vi "Save-Load General Setup Parameters.vi"(8 "error in":errorcluster, 11 "Function":T1=enum."Load from file") -> (0 "error out":errorcluster)   [LabVIEW 2013]
uses:
  Typedefs/Save-Load enum.ctl
  Typedefs/Which path.ctl
  <vilib>/Utility/config.llb/NI_LVConfig.lvlib
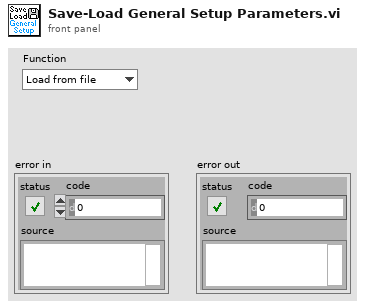
[diagram p1: front panel]
types:
  T1 = typedef "Save-Load enum.ctl" = enum16{"Save to file", "Load from file", "Compare from file"}
  T2 = typedef "Which path.ctl" = enum16{"Configuration Files", "Calibration Files", "Images", "Setup.ini", "Loaded User profile.ini", "User's-Previous session.ini", "New user profile.ini", "Selected User profile.ini", "User profiles folder", "Power meter scaling.txt", "FOV Cal.ini"}
  T3 = typedef "Ini file interface (DBL).ctl" = cluster{"key":string, "Save?":bool, "Default":dbl}[]
  T4 = typedef "Ini file interface (String).ctl" = cluster{"key":string, "Save?":bool, "Default":string}[]
  T5 = typedef "Ini file interface (Boolean).ctl" = cluster{"key":string, "Save?":bool, "Default":bool}[]
  T6 = typedef "NI_LVConfig.lvlib/Config Data RefNum.ctl" = refnum<k1>
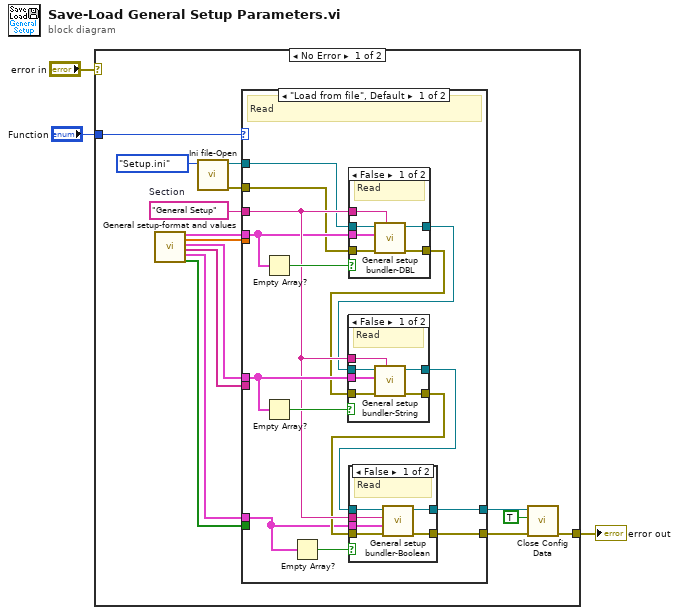
[diagram p0: block diagram]
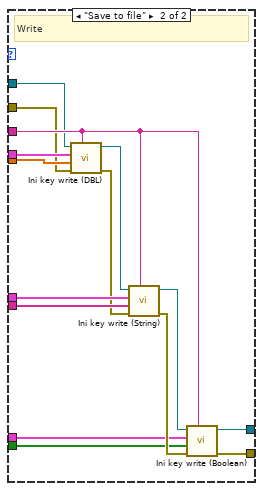
[diagram p5: hidden frame]
diagram:
  n1 = case shown="No Error" "error in" {
    selector: "error in" -> [_ w73]
    tunnel: [w6 w73] -> w3
    tunnel: "Function" -> [w4 _]
    frame No Error {
      w18 = "General Setup"  # Section
      n2 = call "General setup-format and values.vi"() -> ("DBL"=w12:T3, "DBL values"=w11:dbl[], "String"=w10:T4, "String values"=w9:string[], "Boolean"=w8:T5, "Boolean values"=w7:bool[])  [unwired: 14 in]
      n3 = call "Ini file-Open.vi"("Which file?"=Which_path."Setup.ini") -> ("error out"=w15:errorcluster, "User profile ini file ref"=w16:T6)  [unwired: 7 in, 2 out]
      n4 = case shown="\"Load from file\", Default" w4 {
        tunnel: [w31 w63] -> w5
        tunnel: [w32 w62] -> w14
        tunnel: w15 -> [w22 w58]
        tunnel: w16 -> [w23 w59]
        tunnel: w18 -> [w27 w65]
        tunnel: w11 -> [_ w67]
        tunnel: w7 -> [_ w61]
        tunnel: w9 -> [_ w71]
        tunnel: w10 -> [w28 w72]
        tunnel: w12 -> [w24 w68]
        tunnel: w8 -> [w21 w60]
        frame "Load from file", Default {
          # "Read"
          n5 = Empty Array?(array=w24) -> (empty?=w33:bool)
          n6 = Empty Array?(array=w28) -> (empty?=w29:bool)
          n7 = Empty Array?(array=w21) -> (empty?=w30:bool)
          n8 = case shown="False" w33 {
            tunnel: [w54 w57] -> w19
            tunnel: [w55 w56] -> w20
            tunnel: w24 -> [w50 _]
            tunnel: w23 -> [w53 w57]
            tunnel: w22 -> [w52 w56]
            tunnel: w27 -> [w51 _]
            frame False {
              # "Read"
              n9 = call "General setup bundler-DBL.vi"("Section"=w51, "error in (no error)"=w52, "DBL"=w50, "Setup.ini ref"=w53) -> ("error out"=w55:errorcluster, "Setup.ini ref"=w54:T6)  [unwired: 6 in]
            }
            frame True {
              # "No parametersof such type"
            }
          }
          n10 = case shown="False" w29 {
            tunnel: [w38 w41] -> w26
            tunnel: [w37 w40] -> w25
            tunnel: w28 -> [w35 _]
            tunnel: w19 -> [w39 w41]
            tunnel: w20 -> [w36 w40]
            tunnel: w27 -> [w34 _]
            frame False {
              # "Read"
              n11 = call "General setup bundler-String.vi"("Section"=w34, "error in (no error)"=w36, "String"=w35, "Setup.ini ref"=w39) -> ("error out"=w37:errorcluster, "Setup.ini ref"=w38:T6)  [unwired: 6 in]
            }
            frame True {
              # "No parametersof such type"
            }
          }
          n12 = case shown="False" w30 {
            tunnel: [w46 w49] -> w32
            tunnel: [w42 w48] -> w31
            tunnel: w26 -> [w47 w49]
            tunnel: w25 -> [w43 w48]
            tunnel: w27 -> [w45 _]
            tunnel: w21 -> [w44 _]
            frame False {
              # "Read"
              n13 = call "General setup bundler-Boolean.vi"("error in (no error)"=w43, "Boolean"=w44, "Section"=w45, "Setup.ini ref"=w47) -> ("error out"=w42:errorcluster, "Setup.ini ref"=w46:T6)  [unwired: 6 in]
            }
            frame True {
              # "No parametersof such type"
            }
          }
        }
        frame "Save to file" {
          # "Write"
          n14 = call "Ini key write (DBL).vi"("Section"=w65, "error in (no error)"=w58, "Values (DBL)"=w67, "Ini file interface"=w68, "Ini file refnum in"=w59) -> ("error out"=w70:errorcluster, "Ini file refnum out"=w69:T6)  [unwired: 5 in]
          n15 = call "Ini key write (String).vi"("Section"=w65, "error in (no error)"=w70, "Values (String)"=w71, "Ini file interface"=w72, "Ini file refnum in"=w69) -> ("error out"=w64:errorcluster, "Ini file refnum out"=w66:T6)  [unwired: 5 in]
          n16 = call "Ini key write (Boolean).vi"("Section"=w65, "error in (no error)"=w64, "Values (Boolean)"=w61, "Ini file interface"=w60, "Ini file refnum in"=w66) -> ("error out"=w63:errorcluster, "Ini file refnum out"=w62:T6)  [unwired: 5 in]
        }
      }
      n17 = call <vilib>:"Close Config Data.vi"("error in (no error)"=w5, "write file if changed (T)"=TRUE ("write configuration file? (F)"), "refnum"=w14) -> ("error out"=w6:errorcluster)  [unwired: 7 in, 1 out]
    }
    frame Error {
    }
  }
  "error out" <- w3
